vi "Scripting_ConvertSubClassToBaseClass.vi"(0 "SubClass":refnum<vi>, 1 "GOOP4Style":bool, 5 "error in (no error)":errorcluster) -> (19 "error out":errorcluster)   [LabVIEW 2014]
uses:
  <vilib>/Utility/miscctls.llb/LVPositionTypeDef.ctl
  <vilib>/picture/picture.llb/imagedata.ctl
  <resource>/Framework/Providers/Open_GDS/ClassProviders/Provider_EndevoGOOP400/EndevoG4ProviderName.ctl
  <resource>/Framework/Providers/Open_GDS/ClassProviders/Provider_EndevoGOOP400/Templates/EndevoG4TemplateNames.ctl
  <resource>/Framework/Providers/Open_GDS/ClassProviders/Provider_EndevoGOOP300/EndevoProviderName.ctl
  <resource>/Framework/Providers/Open_GDS/ClassProviders/Provider_EndevoGOOP300/Templates/EndevoTemplateNames.ctl
  <resource>/Framework/Providers/Open_GDS/ClassProviders/Provider_LvNativeClass/ClassWriterNative_class/ClassWriterNative.lvclass
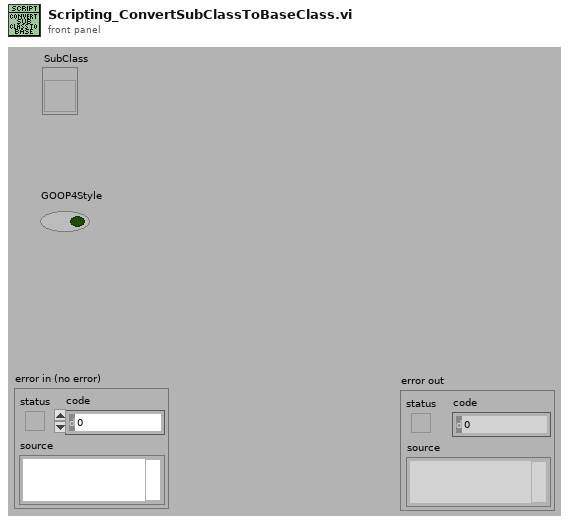
[diagram p1: front panel]
types:
  T1 = cluster{"SubCreate ":path, "ThisSubClass":refnum<vi>, "CurrentBaseClass":refnum<vi>, "SubDestroy":path, "SubKernel":path, "SubAttribute":path, "SubClassAttr":path, "BaseCreate ":path, "BaseDestroy":path, "RootKernel":path, "RootAttribute":path, "RootClassAttr":path, "ThisSubClassName":string, "RootObjectRef":path, "SubObjectRef":path, "AllSubClassFiles":path[], "SubNewVi":path, "ObjectRef":refnum<vi>, "TemplateVersionUsed":string, "BaseNew":path, "Singleton":bool, "AppRef":refnum<vi>}
  T2 = typedef "LVPositionTypeDef.ctl" = cluster{"Left":i32, "Top":i32}
  T3 = typedef "imagedata.ctl" = cluster{"image type":i32, "image depth":i32, "image":u8[], "mask":u8[], "colors":u32[], "Rectangle":cluster{"left":i16, "top":i16, "right":i16, "bottom":i16}}
  T4 = enum32{"invalid VI type", "Standard VI", "Control VI", "Global VI", "Polymorphic VI", "Configuration VI", "SubSystem", "Facade VI", "Method VI"}
  T5 = typedef "EndevoG4TemplateNames.ctl" = enum16{"G4BaseTemplate_Simple_4x4x4", "G4SubTemplate_Simple_4x4x4", "G4BaseTemplate_Simple_6x8x6", "G4SubTemplate_Simple_6x8x6", "G4BaseTemplate_Singleton_4x4x4", "G4SubTemplate_Singleton_4x4x4", "G4BaseTemplate_Singleton_6x8x6", "G4SubTemplate_Singleton_6x8x6", "G4InterfaceTemplate_6x8x6", "G4InterfaceTemplate_4x4x4", "G4BaseTemplate_Simple_5x6x5"}
  T6 = typedef "EndevoG4ProviderName.ctl" = enum16{"EndevoGOOP400"}
  T7 = typedef "EndevoTemplateNames.ctl" = enum16{"BaseTemplate", "SubTemplate", "BaseTemplate_4x4x4", "SubTemplate_4x4x4", "SingletonTemplate"}
  T8 = typedef "EndevoProviderName.ctl" = enum16{"EndevoGOOP300"}
  T9 = typedef "GDSLvCLass_ClassSettingsType.ctl" = cluster{"ClassProviderName":string, "ClassTemplateUsed":string, "ClassTemplateVersion":string, "ClassDescription":string, "PlugIns":T10[], "ConnectorPanePattern":string}
  T10 = typedef "GDSLvClass_PlugIn.ctl" = cluster{"Type":T11, "ID":string, "Version":string, "Path":path, "Name":string, "Data":variant}
  T11 = typedef "GDSLvClass_PlugInTypes.ctl" = enum16{"DesignPattern", "MethodTypes"}
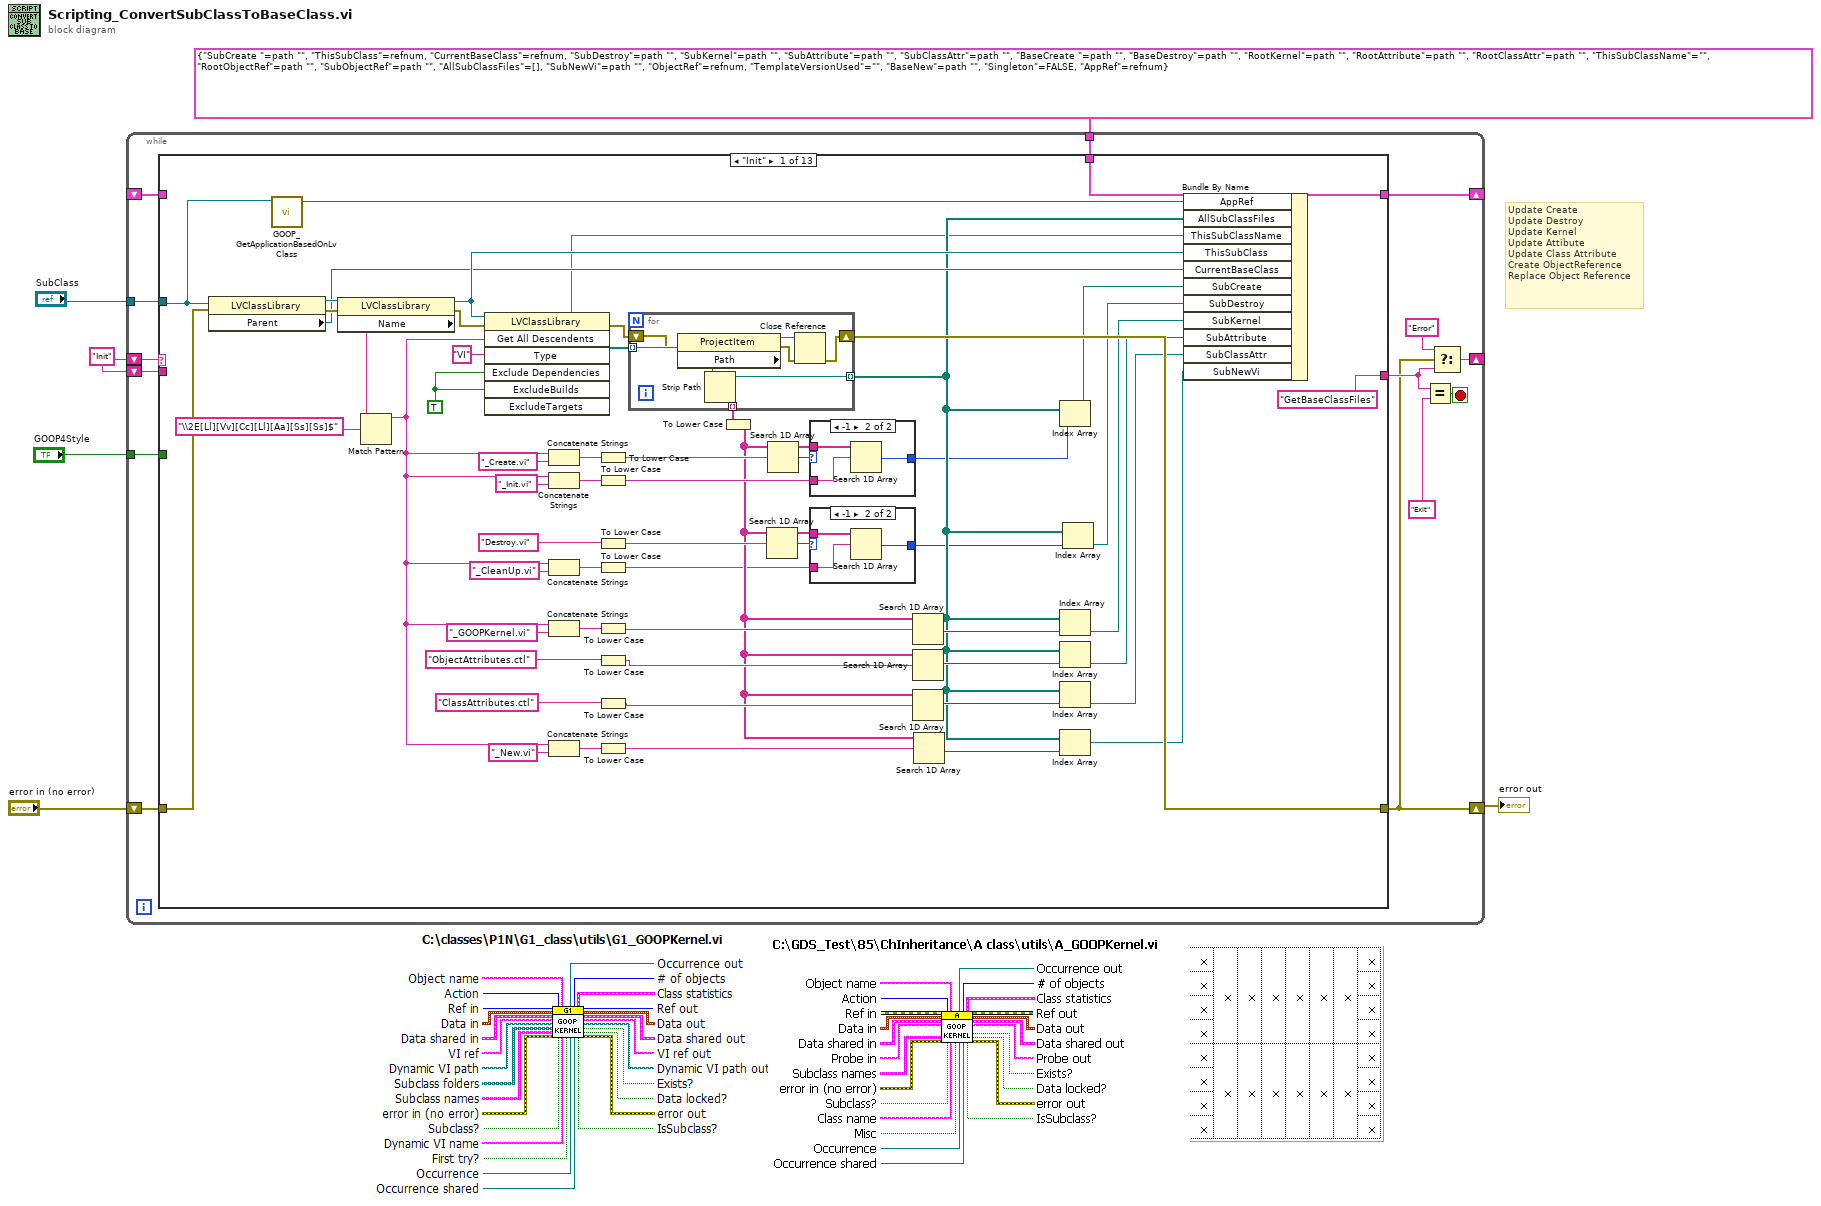
[diagram p0: block diagram]
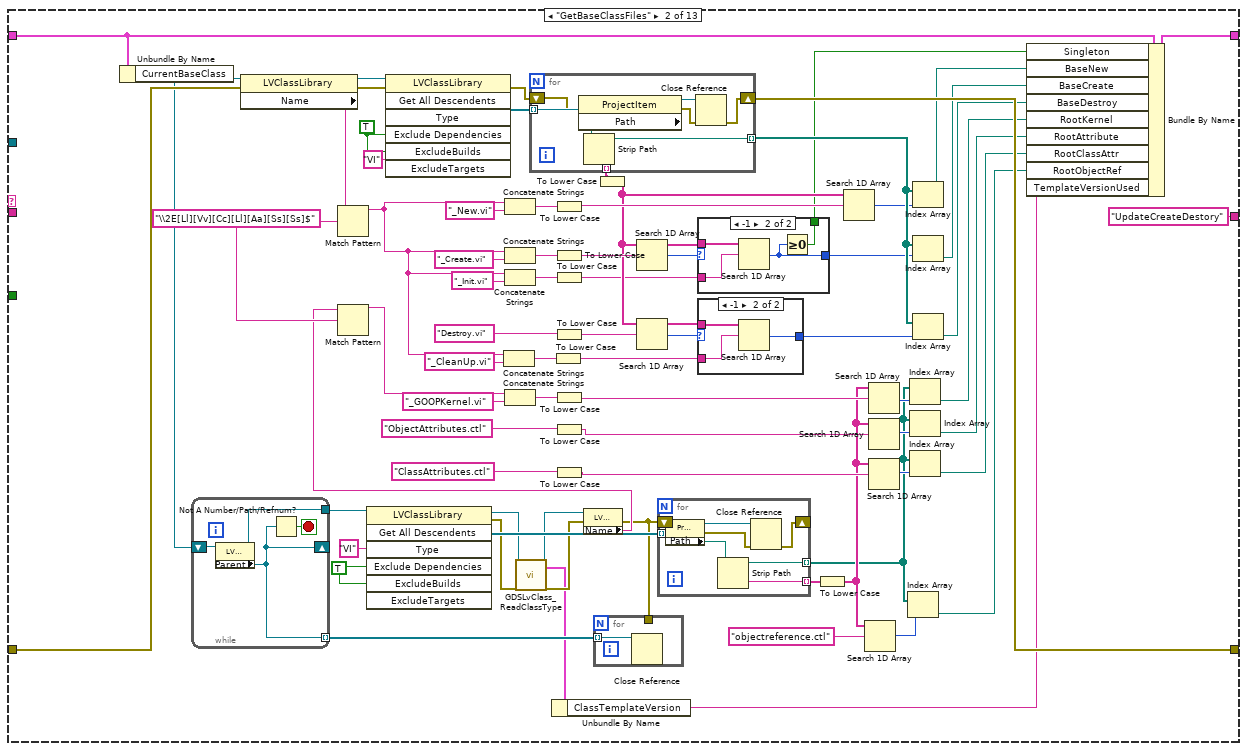
[diagram p4: hidden frame]
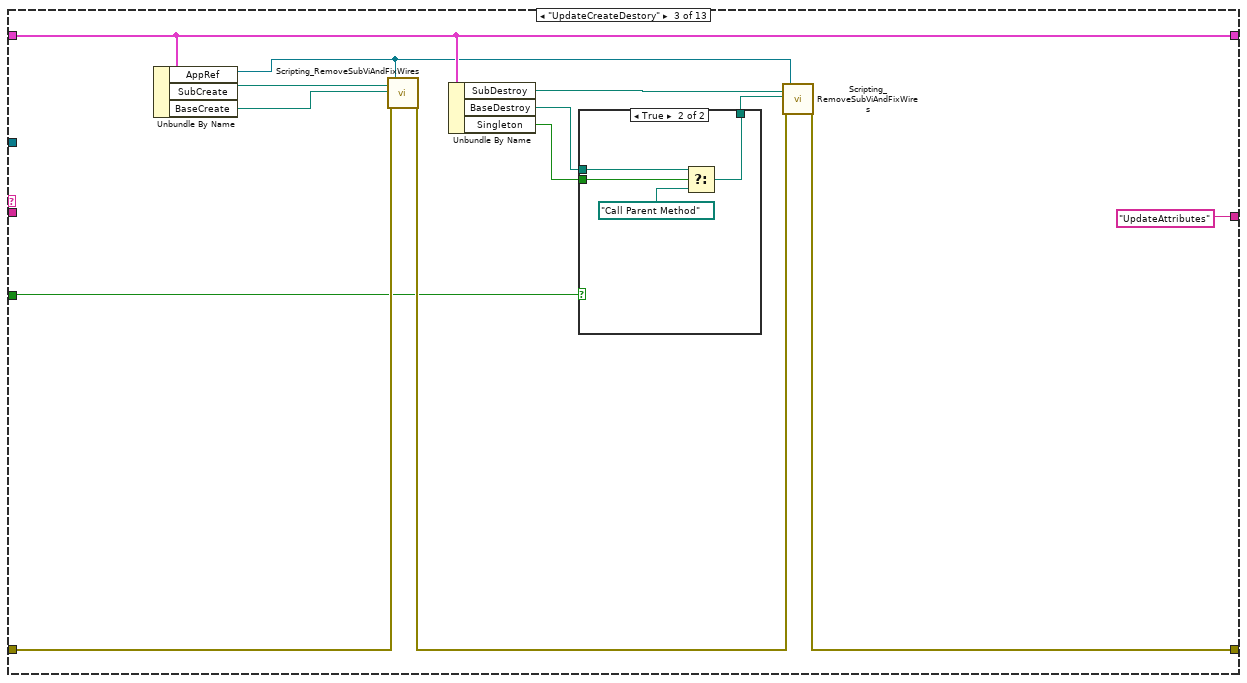
[diagram p7: hidden frame]
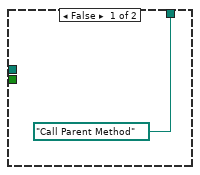
[diagram p8: hidden frame]
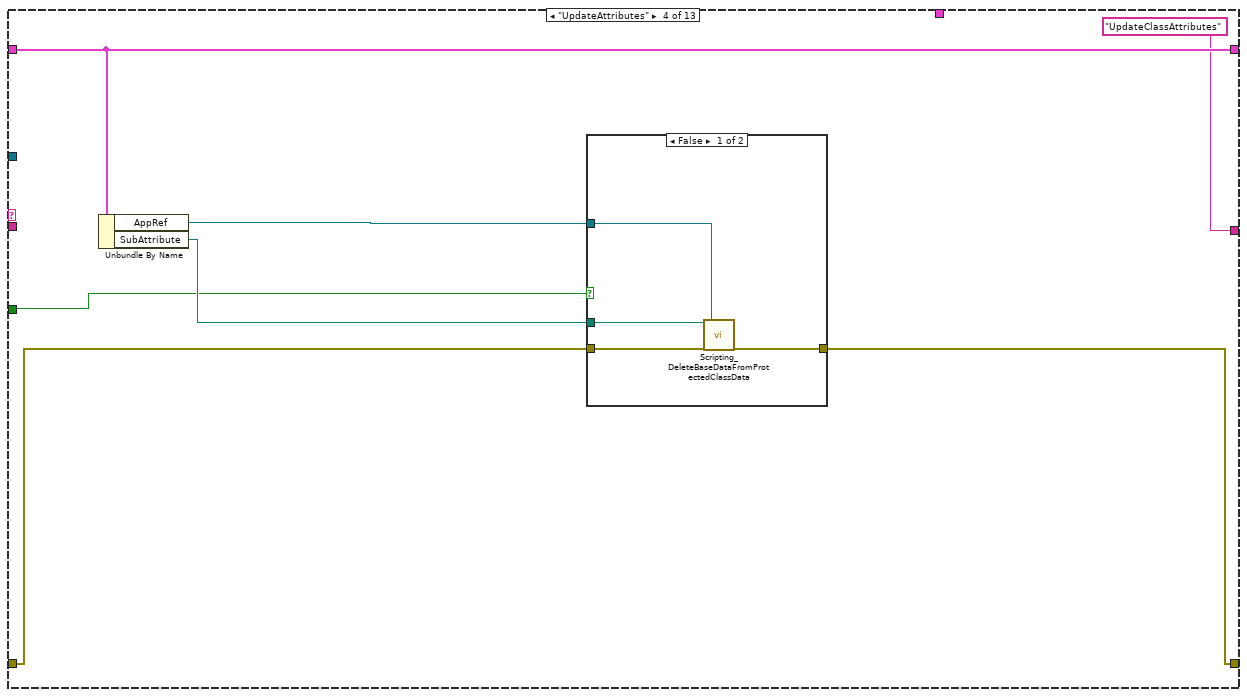
[diagram p9: hidden frame]
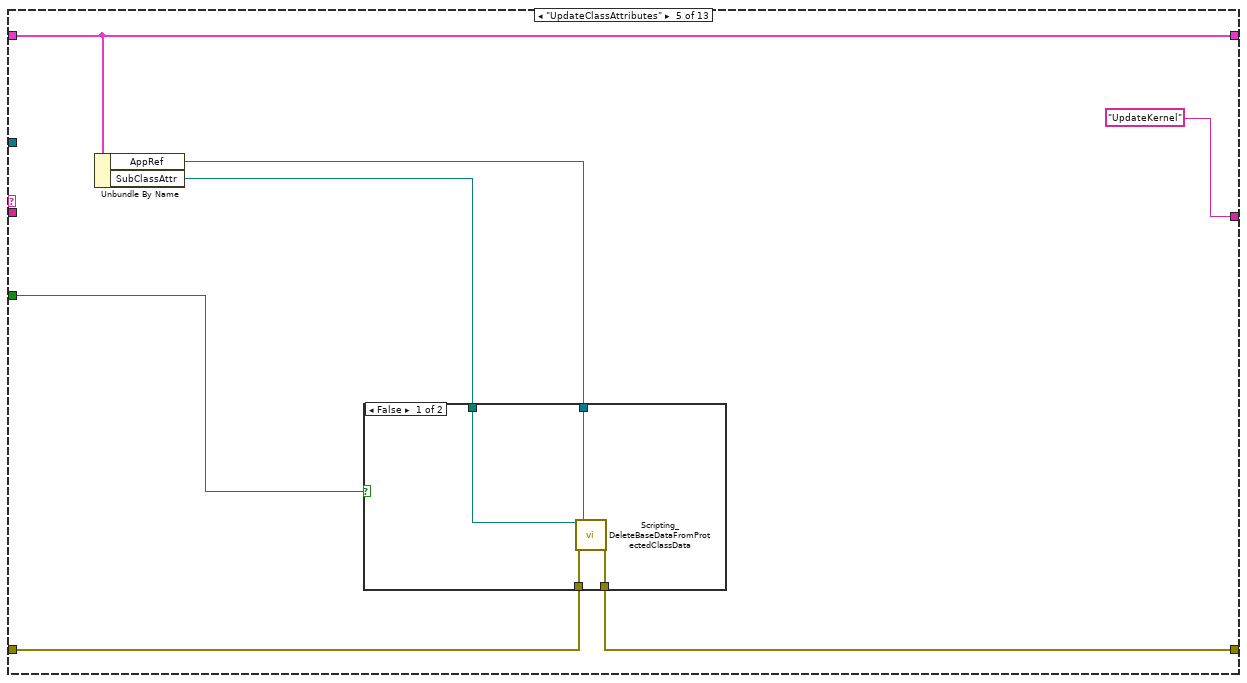
[diagram p11: hidden frame]
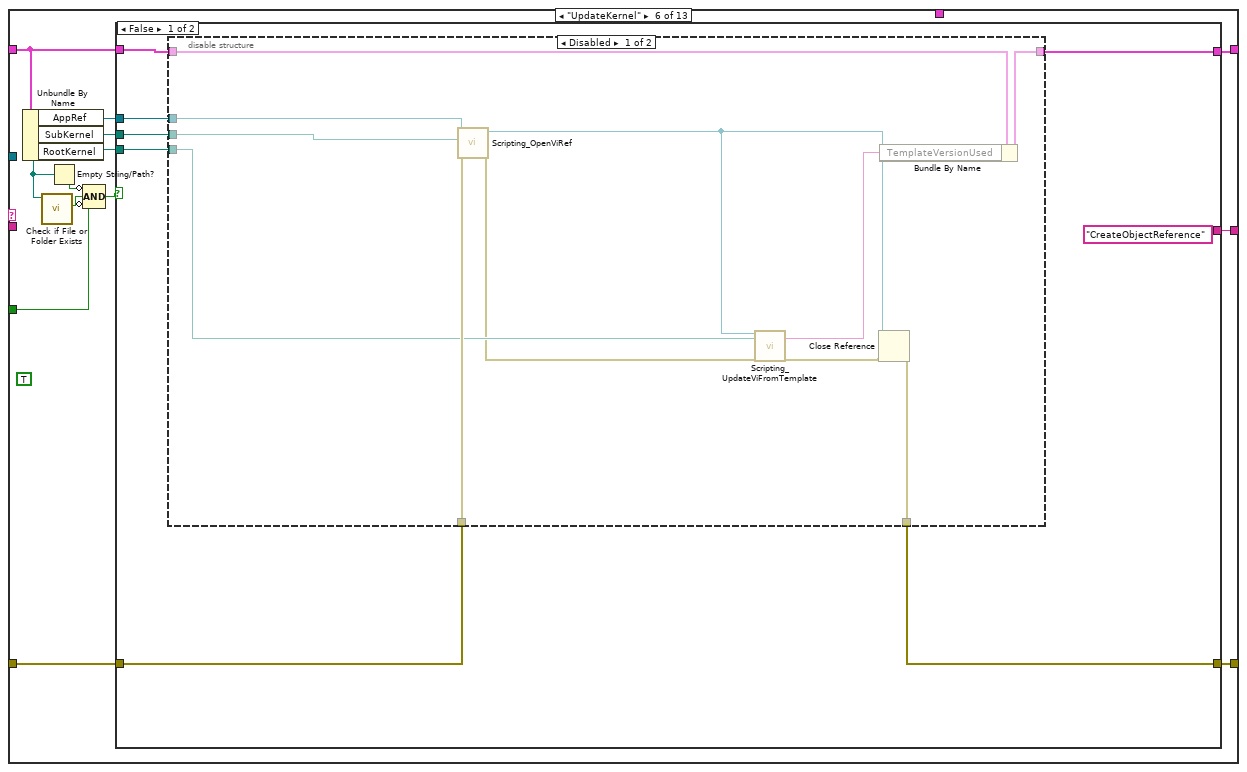
[diagram p13: hidden frame]
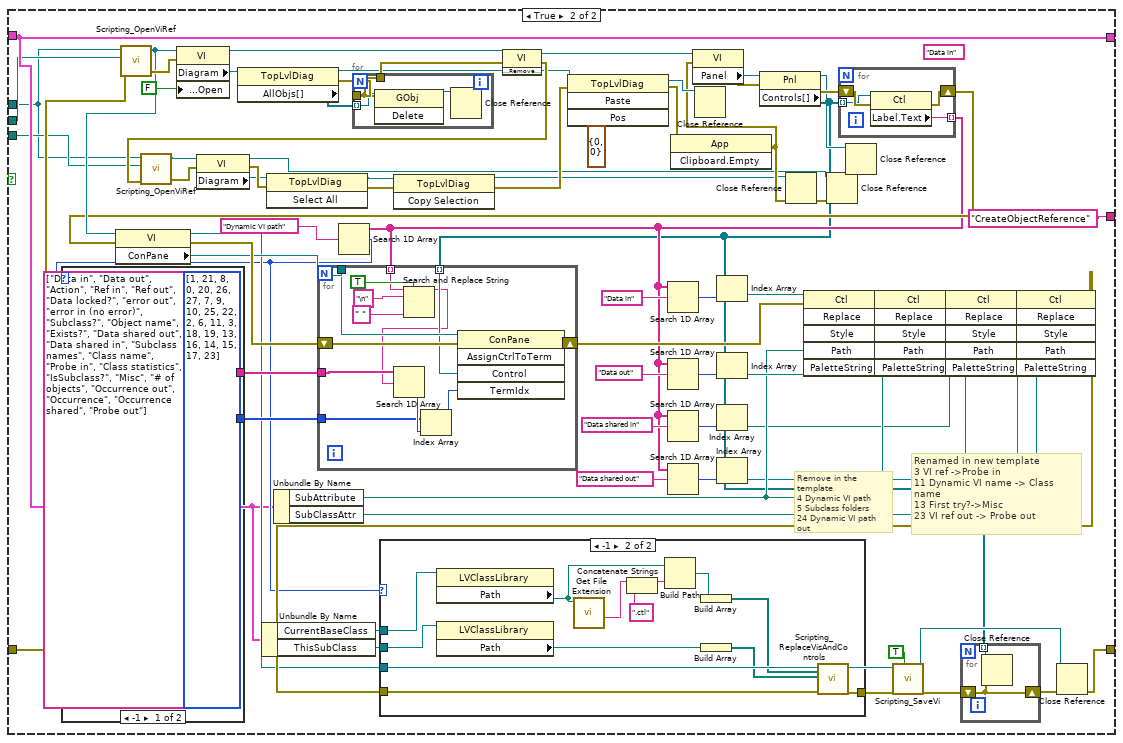
[diagram p15: hidden frame]
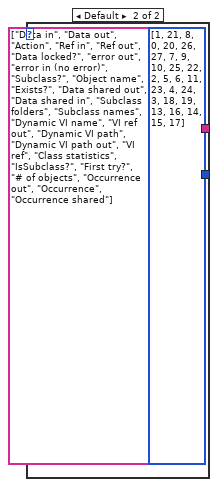
[diagram p17: hidden frame]
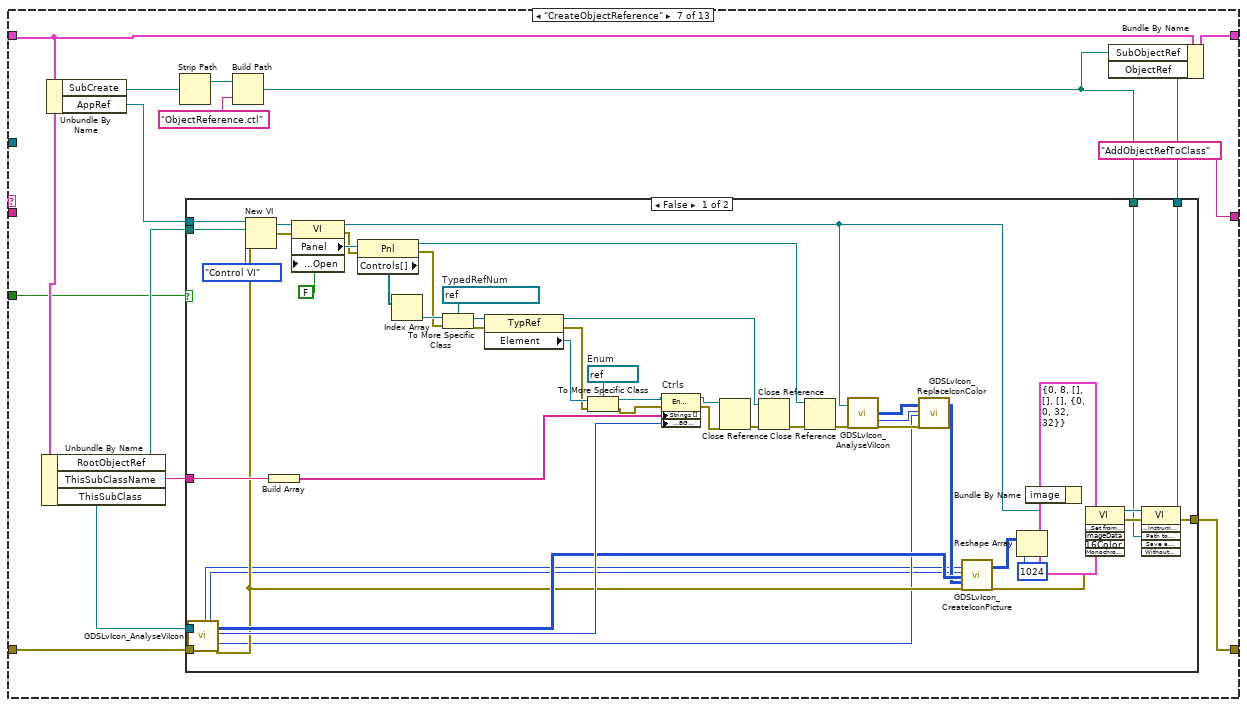
[diagram p18: hidden frame]
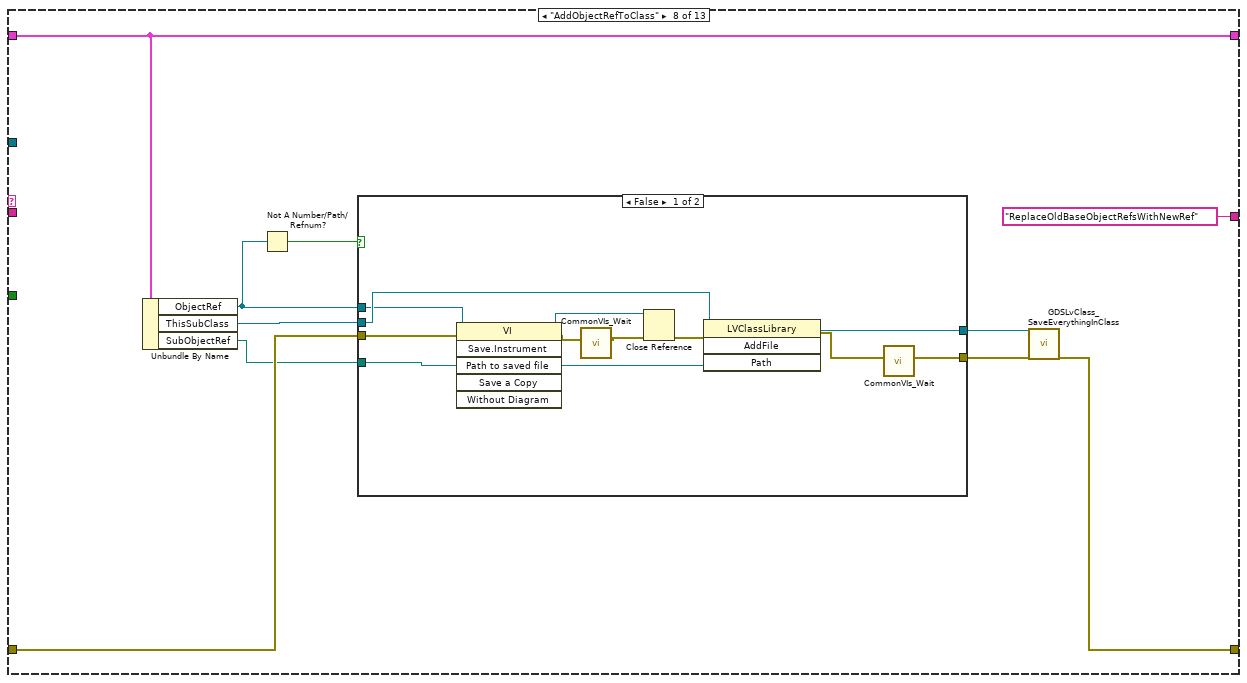
[diagram p20: hidden frame]
diagram:
  w2 = "Init"
  # "Update Create\nUpdate Destroy\nUpdate Kernel\nUpdate Attibute\nUpdate Class Attribute\nCreate ObjectReference\nReplace Object Reference"
  n1 = while {
    shift-right: [w13] -> w5
    shift-left: "error in (no error)" -> [w20]
    shift-right: [w18] -> _
    shift-left: w2 -> [w19]
    shift-right: [w12] -> _
    shift-left: _ -> [w11]
    tunnel: "SubClass" -> [w10]
    tunnel: T1 {"SubCreate "=path "", "ThisSubClass"=refnum, "CurrentBaseClass"=refnum, "SubDestroy"=path "", "SubKernel"=path "", "SubAttribute"=path "", "SubClassAttr"=path "", "BaseCreate "=path "", "BaseDestroy"=path "", "RootKernel"=path "", "RootAttribute"=path "", "RootClassAttr"=path "", "ThisSubClassName"="", "RootObjectRef"=path "", "SubObjectRef"=path "", "AllSubClassFiles"=[], "SubNewVi"=path "", "ObjectRef"=refnum, "TemplateVersionUsed"="", "BaseNew"=path "", "Singleton"=FALSE, "AppRef"=refnum} -> [w9]
    shift-left: w2 -> [w8]
    tunnel: "GOOP4Style" -> [w7]
    stop <- w17 stop-if-true
    n2 = case shown="\"Init\"" w19 {
      tunnel: w20 -> [w45 w136 w204 w218 w229 w247 w390 w457 w485 w538 w578 w588 w597]
      tunnel: [w64 w155 w200 w217 w228 w246 w387 w455 w479 w533 w577 w587 w597] -> w13
      tunnel: ["GetBaseClassFiles" "UpdateCreateDestory" "UpdateAttributes" "UpdateClassAttributes" "UpdateKernel" w248 "AddObjectRefToClass" "ReplaceOldBaseObjectRefsWithNewRef" "RemoveInheritance" "UpdateAllDerivedClasses" "UpdateNEWVI" "CloseReferences" "Exit"] -> w14
      tunnel: [w76 w165 w203 w216 w231 w245 w388 w459 w488 w548 w574 w586 w598] -> w12
      tunnel: w11 -> [_ w137 w203 w216 w231 w244 w385 w459 w488 w548 w574 w586 w598]
      tunnel: w10 -> [w22 _ _ _ _ _ _ _ _ _ w576 _ _]
      tunnel: w9 -> [w44 _ _ _ _ _ _ _ _ _ _ _ _]
      tunnel: w8 -> [_ _ _ _ _ _ _ _ _ _ _ _ w599]
      tunnel: w7 -> [_ _ w198 w214 w226 w238 w383 _ _ w530 w573 w589 _]
      frame "Init" {
        w35 = TRUE ("ExcludeDependencies")
        n3 = property class="LVClassLibrary"(reference=w22, error in=w45) -> (reference out=w72:refnum<vi>, error out=w71:errorcluster, "Parent"=w46:refnum<vi>)
        n4 = call <resource>:"GOOP_GetApplicationBasedOnLvClass.vi"("LVClassLibrary in"=w22) -> ("Application out"=w21:refnum<vi>)  [unwired: 9 in, 1 out]
        n5 = property class="LVClassLibrary"(reference=w72, error in=w71) -> (reference out=w69:refnum<vi>, error out=w70:errorcluster, "Name"=w43:string)
        n6 = Match Pattern(string=w43, regular expression="\\2E[Ll][Vv][Cc][Ll][Aa][Ss][Ss]$") -> (before substring=w25:string)  [unwired: 1 in, 3 out]
        n7 = invoke class="LVClassLibrary" method="Get All Descendents"(reference=w69, error in=w70, "Type"="VI", "Exclude Dependencies"=w35, "ExcludeBuilds"=w35) -> (error out=w73:errorcluster, "All Descendents"=w74:refnum<vi>[])  [unwired: 2 in, 5 out]
        n8 = Concatenate Strings(w25, "_Create.vi" ("string")) -> (w66:string)
        n9 = Concatenate Strings(w25, "_Init.vi" ("string")) -> (w34:string)
        n10 = Concatenate Strings(w25, "_CleanUp.vi" ("string")) -> (w26:string)
        n11 = Concatenate Strings(w25, "_GOOPKernel.vi" ("string")) -> (w60:string)
        n12 = Concatenate Strings(w25, "_New.vi" ("string")) -> (w40:string)
        n13 = To Lower Case(string=w66) -> (all lower case string=w65:string)
        n14 = To Lower Case(string=w34) -> (all lower case string=w31:string)
        n15 = To Lower Case(string="Destroy.vi") -> (all lower case string=w62:string)
        n16 = To Lower Case(string=w26) -> (all lower case string=w23:string)
        n17 = To Lower Case(string=w60) -> (all lower case string=w58:string)
        n18 = To Lower Case(string="ObjectAttributes.ctl") -> (all lower case string=w53:string)
        n19 = To Lower Case(string="ClassAttributes.ctl") -> (all lower case string=w50:string)
        n20 = To Lower Case(string=w40) -> (all lower case string=w41:string)
        n21 = for {
          tunnel: w74 -> [w92] mode=indexing
          shift-right: [w88] -> w64
          shift-left: w73 -> [w89]
          tunnel: [w87] -> w36 mode=indexing
          tunnel: [w86] -> w67 mode=indexing
          n22 = property class="ProjectItem"(reference=w92, error in=w89) -> (reference out=w91:refnum<vi>, error out=w90:errorcluster, "Path"=w87:path)
          n23 = Strip Path(path=w87) -> (name=w86:string)  [unwired: 1 out]
          n24 = Close Reference(reference=w91, error in (no error)=w90) -> (error out=w88:errorcluster)
        }
        n25 = To Lower Case(string=w67) -> (all lower case string=w27:string[])
        n26 = Search 1D Array(1D array=w27, element=w62) -> (index of element=w29:i32)  [unwired: 1 in]
        n27 = Search 1D Array(1D array=w27, element=w65) -> (index of element=w32:i32)  [unwired: 1 in]
        n28 = case shown="-1" w32 {
          selector: w32 -> [w82 _]
          tunnel: w27 -> [_ w85]
          tunnel: w31 -> [_ w84]
          tunnel: [w82 w83] -> w30
          frame 0, Default {
          }
          frame -1 {
            n29 = Search 1D Array(1D array=w85, element=w84) -> (index of element=w83:i32)  [unwired: 1 in]
          }
        }
        n30 = case shown="-1" w29 {
          selector: w29 -> [w78 _]
          tunnel: w27 -> [_ w81]
          tunnel: w23 -> [_ w80]
          tunnel: [w78 w79] -> w28
          frame 0, Default {
          }
          frame -1 {
            n31 = Search 1D Array(1D array=w81, element=w80) -> (index of element=w79:i32)  [unwired: 1 in]
          }
        }
        n32 = Search 1D Array(1D array=w27, element=w58) -> (index of element=w57:i32)  [unwired: 1 in]
        n33 = Search 1D Array(1D array=w27, element=w53) -> (index of element=w52:i32)  [unwired: 1 in]
        n34 = Search 1D Array(1D array=w27, element=w50) -> (index of element=w51:i32)  [unwired: 1 in]
        n35 = Search 1D Array(1D array=w27, element=w41) -> (index of element=w38:i32)  [unwired: 1 in]
        n36 = Index Array(array=w36, index=w30) -> (element=w61:path)
        n37 = Index Array(array=w36, index=w57) -> (element=w49:path)
        n38 = Index Array(array=w36, index=w52) -> (element=w48:path)
        n39 = Index Array(array=w36, index=w51) -> (element=w47:path)
        n40 = Index Array(array=w36, index=w38) -> (element=w37:path)
        n41 = Index Array(array=w36, index=w28) -> (element=w56:path)
        n42 = Bundle By Name(cluster=w44, "AppRef"=w21, "AllSubClassFiles"=w36, "ThisSubClassName"=w25, "ThisSubClass"=w69, "CurrentBaseClass"=w46, "SubCreate"=w61, "SubDestroy"=w56, "SubKernel"=w49, "SubAttribute"=w48, "SubClassAttr"=w47, "SubNewVi"=w37) -> (w76:T1)
      }
      frame "GetBaseClassFiles" {
        w118 = TRUE ("ExcludeDependencies")
        w119 = TRUE ("ExcludeDependencies")
        w128 = "\\2E[Ll][Vv][Cc][Ll][Aa][Ss][Ss]$" ("regular expression")
        n43 = Unbundle By Name(w137) -> ("CurrentBaseClass"=w134:refnum<vi>)
        n44 = while {
          shift-right: [w185] -> _
          shift-left: w134 -> [w186]
          tunnel: [w185] -> w133 mode=indexing
          tunnel: [w184] -> w131
          stop <- w187 stop-if-true
          n45 = property class="LVClassLibrary"(reference=w186) -> (reference out=w184:refnum<vi>, "Parent"=w185:refnum<vi>)  [unwired: 1 in, 1 out]
          n46 = Not A Number/Path/Refnum?(number/path/refnum=w185) -> (NaN/Path/Refnum?=w187:bool)
        }
        n47 = property class="LVClassLibrary"(reference=w134, error in=w136) -> (reference out=w160:refnum<vi>, error out=w161:errorcluster, "Name"=w135:string)
        n48 = Match Pattern(string=w135, regular expression=w128) -> (before substring=w96:string)  [unwired: 1 in, 3 out]
        n49 = invoke class="LVClassLibrary" method="Get All Descendents"(reference=w131, "Type"="VI", "Exclude Dependencies"=w119, "ExcludeBuilds"=w119) -> (reference out=w117:refnum<vi>, error out=w115:errorcluster, "All Descendents"=w130:refnum<vi>[])  [unwired: 3 in, 4 out]
        n50 = invoke class="LVClassLibrary" method="Get All Descendents"(reference=w160, error in=w161, "Type"="VI", "Exclude Dependencies"=w118, "ExcludeBuilds"=w118) -> (error out=w162:errorcluster, "All Descendents"=w163:refnum<vi>[])  [unwired: 2 in, 5 out]
        n51 = Concatenate Strings(w96, "_CleanUp.vi" ("string")) -> (w98:string)
        n52 = Concatenate Strings(w96, "_New.vi" ("string")) -> (w111:string)
        n53 = Concatenate Strings(w96, "_Create.vi" ("string")) -> (w157:string)
        n54 = Concatenate Strings(w96, "_Init.vi" ("string")) -> (w100:string)
        n55 = call <resource>:"GDSLvClass_ReadClassType.vi"("Class Refnum In"=w117, "error in (no error)"=w115) -> ("Class Refnum Out"=w116:refnum<vi>, "ClassSettings"=w113:T9, "error out"=w114:errorcluster)  [unwired: 15 in]
        n56 = for {
          tunnel: w163 -> [w194] mode=indexing
          shift-right: [w190] -> w155
          shift-left: w162 -> [w191]
          tunnel: [w189] -> w108 mode=indexing
          tunnel: [w188] -> w158 mode=indexing
          n57 = property class="ProjectItem"(reference=w194, error in=w191) -> (reference out=w193:refnum<vi>, error out=w192:errorcluster, "Path"=w189:path)
          n58 = Strip Path(path=w189) -> (name=w188:string)  [unwired: 1 out]
          n59 = Close Reference(reference=w193, error in (no error)=w192) -> (error out=w190:errorcluster)
        }
        n60 = Unbundle By Name(w113) -> ("ClassTemplateVersion"=w112:string)
        n61 = To Lower Case(string=w98) -> (all lower case string=w94:string)
        n62 = To Lower Case(string=w111) -> (all lower case string=w109:string)
        n63 = To Lower Case(string=w157) -> (all lower case string=w156:string)
        n64 = To Lower Case(string=w100) -> (all lower case string=w95:string)
        n65 = To Lower Case(string="Destroy.vi") -> (all lower case string=w153:string)
        n66 = To Lower Case(string="ObjectAttributes.ctl") -> (all lower case string=w144:string)
        n67 = To Lower Case(string="ClassAttributes.ctl") -> (all lower case string=w141:string)
        n68 = property class="LVClassLibrary"(reference=w116, error in=w114) -> (error out=w120:errorcluster, "Name"=w126:string)  [unwired: 1 out]
        n69 = Match Pattern(string=w126, regular expression=w128) -> (before substring=w127:string)  [unwired: 1 in, 3 out]
        n70 = Concatenate Strings(w127, "_GOOPKernel.vi" ("string")) -> (w151:string)
        n71 = To Lower Case(string=w151) -> (all lower case string=w149:string)
        n72 = for {
          tunnel: w133 -> [w183] mode=indexing
          tunnel: w120 -> [_]
          n73 = Close Reference(reference=w183) -> ()  [unwired: 1 in, 1 out]
        }
        n74 = To Lower Case(string=w158) -> (all lower case string=w101:string[])
        n75 = Search 1D Array(1D array=w101, element=w156) -> (index of element=w104:i32)  [unwired: 1 in]
        n76 = Search 1D Array(1D array=w101, element=w153) -> (index of element=w105:i32)  [unwired: 1 in]
        n77 = for {
          tunnel: w130 -> [w182] mode=indexing
          shift-right: [w178] -> _
          shift-left: w120 -> [w179]
          tunnel: [w177] -> w122 mode=indexing
          tunnel: [w176] -> w129 mode=indexing
          n78 = property class="ProjectItem"(reference=w182, error in=w179) -> (reference out=w181:refnum<vi>, error out=w180:errorcluster, "Path"=w177:path)
          n79 = Strip Path(path=w177) -> (name=w176:string)  [unwired: 1 out]
          n80 = Close Reference(reference=w181, error in (no error)=w180) -> (error out=w178:errorcluster)
        }
        n81 = case shown="-1" w104 {
          selector: w104 -> [w171 _]
          tunnel: w101 -> [_ w175]
          tunnel: w95 -> [_ w174]
          tunnel: [w171 w173] -> w103
          tunnel: [_ w172] -> w93
          frame 0, Default {
          }
          frame -1 {
            n82 = Search 1D Array(1D array=w175, element=w174) -> (index of element=w173:i32)  [unwired: 1 in]
            n83 = Greater Or Equal To 0?(x=w173) -> (x >= 0?=w172:bool)
          }
        }
        n84 = case shown="-1" w105 {
          selector: w105 -> [w167 _]
          tunnel: w101 -> [_ w170]
          tunnel: w94 -> [_ w169]
          tunnel: [w167 w168] -> w102
          frame 0, Default {
          }
          frame -1 {
            n85 = Search 1D Array(1D array=w170, element=w169) -> (index of element=w168:i32)  [unwired: 1 in]
          }
        }
        n86 = To Lower Case(string=w129) -> (all lower case string=w123:string[])
        n87 = Search 1D Array(1D array=w101, element=w109) -> (index of element=w107:i32)  [unwired: 1 in]
        n88 = Search 1D Array(1D array=w123, element="objectreference.ctl") -> (index of element=w124:i32)  [unwired: 1 in]
        n89 = Search 1D Array(1D array=w123, element=w149) -> (index of element=w148:i32)  [unwired: 1 in]
        n90 = Search 1D Array(1D array=w123, element=w144) -> (index of element=w143:i32)  [unwired: 1 in]
        n91 = Search 1D Array(1D array=w123, element=w141) -> (index of element=w142:i32)  [unwired: 1 in]
        n92 = Index Array(array=w122, index=w124) -> (element=w121:path)
        n93 = Index Array(array=w122, index=w148) -> (element=w140:path)
        n94 = Index Array(array=w122, index=w143) -> (element=w139:path)
        n95 = Index Array(array=w122, index=w142) -> (element=w138:path)
        n96 = Index Array(array=w108, index=w107) -> (element=w106:path)
        n97 = Index Array(array=w108, index=w103) -> (element=w152:path)
        n98 = Index Array(array=w108, index=w102) -> (element=w147:path)
        n99 = Bundle By Name(cluster=w137, "Singleton"=w93, "BaseNew"=w106, "BaseCreate"=w152, "BaseDestroy"=w147, "RootKernel"=w140, "RootAttribute"=w139, "RootClassAttr"=w138, "RootObjectRef"=w121, "TemplateVersionUsed"=w112) -> (w165:T1)
      }
      frame "UpdateCreateDestory" {
        n100 = Unbundle By Name(w203) -> ("AppRef"=w195:refnum<vi>, "SubCreate"=w206:path, "BaseCreate"=w205:path)
        n101 = call <resource>:"Scripting_RemoveSubViAndFixWires.vi"("MainViPath/ViRef/BlockDiagramRef"=w206, "SubVIToRemove"=w205, "error in (no error)"=w204, "AppRef"=w195) -> ("error out"=w201:errorcluster)  [unwired: 15 in]
        n102 = Unbundle By Name(w203) -> ("SubDestroy"=w202:path, "BaseDestroy"=w196:path, "Singleton"=w197:bool)
        n103 = case shown="True" w198 {
          tunnel: [path "Call Parent Method" ("SubVIToRemove") w209] -> w199
          tunnel: w197 -> [_ w212]
          tunnel: w196 -> [_ w210]
          frame False {
          }
          frame True {
            n104 = Select(t=w210, s=w212, f=path "Call Parent Method" ("SubVIToRemove")) -> (s? t:f=w209:path)
          }
        }
        n105 = call <resource>:"Scripting_RemoveSubViAndFixWires.vi"("MainViPath/ViRef/BlockDiagramRef"=w202, "SubVIToRemove"=w199, "error in (no error)"=w201, "AppRef"=w195) -> ("error out"=w200:errorcluster)  [unwired: 15 in]
      }
      frame "UpdateAttributes" {
        n106 = Unbundle By Name(w216) -> ("AppRef"=w213:refnum<vi>, "SubAttribute"=w219:path)
        n107 = case shown="False" w214 {
          tunnel: w219 -> [w223 _]
          tunnel: w218 -> [w222 w224]
          tunnel: [w221 w224] -> w217
          tunnel: w213 -> [w220 _]
          frame False {
            n108 = call <resource>:"Scripting_DeleteBaseDataFromProtectedClassData.vi"("SubAttribute"=w223, "error in (no error)"=w222, "AppRef"=w220) -> ("error out"=w221:errorcluster)  [unwired: 16 in]
          }
          frame True {
          }
        }
      }
      frame "UpdateClassAttributes" {
        n109 = Unbundle By Name(w231) -> ("AppRef"=w225:refnum<vi>, "SubClassAttr"=w227:path)
        n110 = case shown="False" w226 {
          tunnel: w229 -> [w235 w236]
          tunnel: [w234 w236] -> w228
          tunnel: w227 -> [w233 _]
          tunnel: w225 -> [w232 _]
          frame False {
            n111 = call <resource>:"Scripting_DeleteBaseDataFromProtectedClassData.vi"("SubAttribute"=w233, "error in (no error)"=w235, "AppRef"=w232) -> ("error out"=w234:errorcluster)  [unwired: 16 in]
          }
          frame True {
          }
        }
      }
      frame "UpdateKernel" {
        (unwired) TRUE
        n112 = Unbundle By Name(w244) -> ("AppRef"=w237:refnum<vi>, "SubKernel"=w242:path, "RootKernel"=w243:path)
        n113 = call <vilib>:"Check if File or Folder Exists.vi"("path"=w242) -> ("file or folder exists?"=w239:bool)  [unwired: 8 in, 2 out]
        n114 = Empty String/Path?(string/path=w242) -> (empty?=w241:bool)
        n115 = Compound Arithmetic op=AND(invert w241, w239, invert w238) -> (w240:bool)
        n116 = case shown="False" w240 {
          tunnel: ["CreateObjectReference" "CreateObjectReference"] -> w248
          tunnel: w247 -> [w253 w315]
          tunnel: w244 -> [w255 w275]
          tunnel: [w252 w283] -> w246
          tunnel: [w254 w275] -> w245
          tunnel: w242 -> [w251 w272]
          tunnel: w243 -> [w250 w271]
          tunnel: w237 -> [w249 w270]
          frame False {
            n117 = disable-structure shown="Disabled" {
              disable-tunnel: w255 -> [w266 w268]
              disable-tunnel: [w265 w268] -> w254
              disable-tunnel: w253 -> [w264 w269]
              disable-tunnel: [w263 w269] -> w252
              disable-tunnel: w251 -> [w262 _]
              disable-tunnel: w250 -> [w261 _]
              disable-tunnel: w249 -> [w257 _]
              frame Disabled {
                n118 = call <resource>:"Scripting_OpenViRef.vi"("error in"=w264, "ViPath/ViName/Viref"=w262, "AppRef"=w257) -> ("error out"=w260:errorcluster, "vi reference"=w258:refnum<vi>)  [unwired: 6 in, 1 out]
                n119 = call <resource>:"Scripting_UpdateViFromTemplate.vi"("ViRef"=w258, "TemplateVI(Path or Ref)"=w261, "error in (no error)"=w260) -> ("TemplateVersionUsed"=w267:string, "error out"=w259:errorcluster)  [unwired: 15 in]
                n120 = Close Reference(reference=w258, error in (no error)=w259) -> (error out=w263:errorcluster)
                n121 = Bundle By Name(cluster=w266, "TemplateVersionUsed"=w267) -> (w265:T1)
              }
              frame Enabled {
              }
            }
          }
          frame True {
            (unwired) "Data in" ("Label.Text")
            # "Renamed in new template\n3 VI ref ->Probe in\n11 Dynamic VI name -> Class name\n13 First try?->Misc\n23 VI ref out -> Probe out"
            # "Remove in the template\n4 Dynamic VI path\n5 Subclass folders\n24 Dynamic VI path out"
            n122 = call <resource>:"Scripting_OpenViRef.vi"("error in"=w315, "ViPath/ViName/Viref"=w272, "AppRef"=w270) -> ("error out"=w340:errorcluster, "vi reference"=w329:refnum<vi>)  [unwired: 6 in, 1 out]
            n123 = property class="VI"(reference=w329, error in=w340, "Front Panel.Open"=FALSE ("Front Panel Window:Open")) -> (reference out=w324:refnum<vi>, "Diagram"=w327:refnum<vi>)  [unwired: 1 out]
            n124 = property class="TopLvlDiag"(reference=w327) -> (reference out=w320:refnum<vi>, error out=w326:errorcluster, "AllObjs[]"=w325:refnum<vi>[])  [unwired: 1 in]
            n125 = Unbundle By Name(w275) -> ("CurrentBaseClass"=w274:refnum<vi>, "ThisSubClass"=w273:refnum<vi>)
            n126 = Unbundle By Name(w275) -> ("SubAttribute"=w302:path, "SubClassAttr"=w297:path)
            n127 = for {
              tunnel: w326 -> [w375]
              tunnel: w325 -> [w376] mode=indexing
              tunnel: [w375] -> w323
              n128 = invoke class="GObj" method="Delete"(reference=w376, error in=w375) -> (reference out=w377:refnum<vi>)  [unwired: 1 in, 2 out]
              n129 = Close Reference(reference=w377) -> ()  [unwired: 1 in, 1 out]
            }
            n130 = invoke class="VI" method="BD.Remove Bad Wires"(reference=w324, error in=w323) -> (reference out=w319:refnum<vi>, error out=w322:errorcluster)  [unwired: 1 in, 1 out]
            n131 = call <resource>:"Scripting_OpenViRef.vi"("error in"=w322, "ViPath/ViName/Viref"=w271, "AppRef"=w270) -> ("error out"=w335:errorcluster, "vi reference"=w334:refnum<vi>)  [unwired: 6 in, 1 out]
            n132 = property class="VI"(reference=w334, error in=w335) -> (reference out=w290:refnum<vi>, error out=w339:errorcluster, "Diagram"=w336:refnum<vi>)
            n133 = invoke class="TopLvlDiag" method="Select All"(reference=w336, error in=w339) -> (reference out=w337:refnum<vi>, error out=w338:errorcluster)  [unwired: 1 in, 1 out]
            n134 = invoke class="TopLvlDiag" method="Copy Selection"(reference=w337, error in=w338) -> (reference out=w292:refnum<vi>, error out=w321:errorcluster)  [unwired: 1 in, 1 out]
            n135 = invoke class="TopLvlDiag" method="Paste"(reference=w320, error in=w321, "Pos"=T2 {"Left"=0, "Top"=0} ("Position")) -> (reference out=w295:refnum<vi>, error out=w296:errorcluster)  [unwired: 1 in, 2 out]
            n136 = invoke class="App" method="Clipboard.Empty"(error in=w296) -> (error out=w293:errorcluster)  [unwired: 2 in, 2 out]
            n137 = property class="VI"(reference=w319, error in=w293) -> (error out=w331:errorcluster, "Panel"=w332:refnum<vi>)  [unwired: 1 out]
            n138 = Close Reference(reference=w295) -> ()  [unwired: 1 in, 1 out]
            n139 = property class="Pnl"(reference=w332, error in=w331) -> (reference out=w294:refnum<vi>, error out=w330:errorcluster, "Controls[]"=w280:refnum<vi>[])
            n140 = Close Reference(reference=w292, error in (no error)=w293) -> (error out=w291:errorcluster)
            n141 = Close Reference(reference=w290, error in (no error)=w291) -> ()  [unwired: 1 out]
            n142 = for {
              tunnel: w280 -> [w378] mode=indexing
              shift-right: [w380] -> w328
              shift-left: w330 -> [w381]
              tunnel: [w379] -> w285 mode=indexing
              n143 = property class="Ctl"(reference=w378, error in=w381) -> (error out=w380:errorcluster, "Label.Text"=w379:string)  [unwired: 1 out]
            }
            n144 = property class="VI"(reference=w329, error in=w328) -> (reference out=w277:refnum<vi>, error out=w316:errorcluster, "ConPane"=w282:refnum<vi>)
            n145 = Search 1D Array(1D array=w285, element="Dynamic VI path" ("Id")) -> (index of element=w276:i32)  [unwired: 1 in]
            n146 = case shown="-1" w276 {
              tunnel: [string[] ["Data in", "Data out", "Action", "Ref in", "Ref out", "Data locked?", "error out", "error in (no error)", "Subclass?", "Object name", "Exists?", "Data shared out", "Data shared in", "Subclass names", "Class name", "Probe in", "Class statistics", "IsSubclass?", "Misc", "# of objects", "Occurrence out", "Occurrence", "Occurrence shared", "Probe out"] ("Array") string[] ["Data in", "Data out", "Action", "Ref in", "Ref out", "Data locked?", "error out", "error in (no error)", "Subclass?", "Object name", "Exists?", "Data shared out", "Data shared in", "Subclass folders", "Subclass names", "Dynamic VI name", "VI ref out", "Dynamic VI path", "Dynamic VI path out", "VI ref", "Class statistics", "IsSubclass?", "First try?", "# of objects", "Occurrence out", "Occurrence", "Occurrence shared"] ("Array")] -> w318
              tunnel: [i32[] [1, 21, 8, 0, 20, 26, 27, 7, 9, 10, 25, 22, 2, 6, 11, 3, 18, 19, 13, 16, 14, 15, 17, 23] i32[] [1, 21, 8, 0, 20, 26, 27, 7, 9, 10, 25, 22, 2, 5, 6, 11, 23, 4, 24, 3, 18, 19, 13, 16, 14, 15, 17]] -> w317
              frame -1 {
              }
              frame Default {
              }
            }
            n147 = for {
              tunnel: w285 -> [w361] mode=indexing
              tunnel: w282 -> [w372]
              tunnel: w318 -> [w365]
              tunnel: w280 -> [w366] mode=indexing
              tunnel: w317 -> [w370]
              shift-right: [w367] -> w310
              shift-left: w316 -> [w368]
              n148 = Search and Replace String(replace all?=TRUE ("replace all? (F)"), input string=w361, search string="\n", replace string=" " ("replace string (\"\")")) -> (result string=w360:string)  [unwired: 4 in, 3 out]
              n149 = Search 1D Array(1D array=w365, element=w360) -> (index of element=w371:i32)  [unwired: 1 in]
              n150 = Index Array(array=w370, index=w371) -> (element=w369:i32)
              n151 = invoke class="ConPane" method="AssignCtrlToTerm"(reference=w372, error in=w368, "Control"=w366, "TermIdx"=w369) -> (error out=w367:errorcluster)  [unwired: 1 in, 4 out]
            }
            n152 = Search 1D Array(1D array=w285, element="Data in" ("Label.Text")) -> (index of element=w314:i32)  [unwired: 1 in]
            n153 = Search 1D Array(1D array=w285, element="Data out" ("Label.Text")) -> (index of element=w309:i32)  [unwired: 1 in]
            n154 = Search 1D Array(1D array=w285, element="Data shared in" ("Label.Text")) -> (index of element=w308:i32)  [unwired: 1 in]
            n155 = Search 1D Array(1D array=w285, element="Data shared out" ("Label.Text")) -> (index of element=w307:i32)  [unwired: 1 in]
            n156 = Index Array(array=w280, index=w314) -> (element=w312:refnum<vi>)
            n157 = Index Array(array=w280, index=w309) -> (element=w303:refnum<vi>)
            n158 = Index Array(array=w280, index=w308) -> (element=w299:refnum<vi>)
            n159 = Index Array(array=w280, index=w307) -> (element=w298:refnum<vi>)
            n160 = invoke class="Ctl" method="Replace"(reference=w312, error in=w310, "Path"=w302) -> (error out=w311:errorcluster)  [unwired: 3 in, 5 out]
            n161 = Close Reference(reference=w294) -> ()  [unwired: 1 in, 1 out]
            n162 = invoke class="Ctl" method="Replace"(reference=w303, error in=w311, "Path"=w302) -> (error out=w300:errorcluster)  [unwired: 3 in, 5 out]
            n163 = invoke class="Ctl" method="Replace"(reference=w299, error in=w300, "Path"=w297) -> (error out=w301:errorcluster)  [unwired: 3 in, 5 out]
            n164 = invoke class="Ctl" method="Replace"(reference=w298, error in=w301, "Path"=w297) -> (error out=w279:errorcluster)  [unwired: 3 in, 5 out]
            n165 = case shown="-1" w276 {
              tunnel: w277 -> [_ w355]
              tunnel: w279 -> [w342 w354]
              tunnel: [w342 w353] -> w278
              tunnel: w274 -> [_ w350]
              tunnel: w273 -> [_ w349]
              frame Default {
              }
              frame -1 {
                n166 = property class="LVClassLibrary"(reference=w350) -> ("Path"=w346:path)  [unwired: 1 in, 2 out]
                n167 = property class="LVClassLibrary"(reference=w349) -> ("Path"=w348:path)  [unwired: 1 in, 2 out]
                n168 = call <vilib>:"Get File Extension.vi"("file"=w346) -> ("filename without extension"=w345:string)  [unwired: 7 in, 3 out]
                n169 = Concatenate Strings(w345, ".ctl" ("string")) -> (w344:string)
                n170 = Build Path(base path=w346, name or relative path=w344) -> (appended path=w347:path)
                n171 = Build Array(w347) -> (w352:path[])
                n172 = Build Array(w348) -> (w351:path[])
                n173 = call <resource>:"Scripting_ReplaceVisAndControls.vi"("ViRef"=w355, "OldVIsAndControls"=w352, "NewVIsAndControls"=w351, "error in (no error)"=w354) -> ("error out"=w353:errorcluster)  [unwired: 14 in, 1 out]
              }
            }
            n174 = call <resource>:"Scripting_SaveVi.vi"("ForceResaving(False)"=TRUE, "error in (no error)"=w278, "VIRefToSaveIn"=w277) -> ("error out"=w287:errorcluster, "VIRefToSaveOut"=w288:refnum<vi>)  [unwired: 7 in]
            n175 = for {
              tunnel: w280 -> [w374] mode=indexing
              shift-right: [w373] -> w289
              shift-left: w287 -> [w373]
              n176 = Close Reference(reference=w374, error in (no error)=w373) -> ()  [unwired: 1 out]
            }
            n177 = Close Reference(reference=w288, error in (no error)=w289) -> (error out=w283:errorcluster)
          }
        }
      }
      frame "CreateObjectReference" {
        n178 = Unbundle By Name(w385) -> ("RootObjectRef"=w391:path, "ThisSubClassName"=w394:string, "ThisSubClass"=w389:refnum<vi>)
        n179 = Unbundle By Name(w385) -> ("SubCreate"=w393:path, "AppRef"=w382:refnum<vi>)
        n180 = Strip Path(path=w393) -> (stripped path=w396:path)  [unwired: 1 out]
        n181 = Build Path(base path=w396, name or relative path="ObjectReference.ctl") -> (appended path=w384:path)
        n182 = case shown="False" w383 {
          tunnel: w394 -> [w446 _]
          tunnel: w391 -> [w445 _]
          tunnel: w390 -> [w414 w449]
          tunnel: w389 -> [w413 _]
          tunnel: [w400 w449] -> w387
          tunnel: [w399 _] -> w386
          tunnel: w384 -> [w398 _]
          tunnel: w382 -> [w397 _]
          frame False {
            w434 = refnum<vi> refnum  # Enum
            w439 = refnum<vi> refnum  # TypedRefNum
            n183 = call <resource>:"GDSLvIcon_AnalyseViIcon.vi"("ViRef/LvCLassRef/LvLibRef/ViPath"=w413, "error in (no error)"=w414) -> ("FrameColor"=w403:u32, "FrameThickness(1)"=w402:u32, "HeaderIcon"=w411:u8[][], "HeaderBkColor"=w412:u32, "BodyBkColor"=w404:u32, "error out"=w409:errorcluster)  [unwired: 5 in, 7 out]
            n184 = New VI(8:w409, 9:T4."Control VI" ("vi type (standard vi)"), 10:w445, 11:w397) -> (0:w448:errorcluster, 3:w447:refnum<vi>)  [unwired: 3 in]
            n185 = Build Array(w446) -> (w425:string[])
            n186 = property class="VI"(reference=w447, error in=w448, "Front Panel.Open"=FALSE ("Front Panel Window:Open")) -> (reference out=w401:refnum<vi>, error out=w435:errorcluster, "Panel"=w442:refnum<vi>)
            n187 = property class="Pnl"(reference=w442, error in=w435) -> (reference out=w429:refnum<vi>, error out=w436:errorcluster, "Controls[]"=w441:refnum<vi>[])
            n188 = Index Array(array=w441) -> (element=w440:refnum<vi>)  [unwired: 1 in]
            n189 = To More Specific Class(target class=w439, reference=w440, error in=w436) -> (specific class reference=w437:refnum<vi>, error out=w438:errorcluster)
            n190 = property class="TypRef"(reference=w437, error in=w438) -> (reference out=w431:refnum<vi>, error out=w432:errorcluster, "Element"=w433:refnum<vi>)
            n191 = To More Specific Class(target class=w434, reference=w433, error in=w432) -> (specific class reference=w427:refnum<vi>, error out=w426:errorcluster)
            n192 = property on="Ctrls" class="Enum"(reference=w427, error in=w426, "Strings []"=w425, "Named Numeric Colors:BG Color"=w412) -> (reference out=w424:refnum<vi>, error out=w423:errorcluster)
            n193 = Close Reference(reference=w424, error in (no error)=w423) -> (error out=w443:errorcluster)
            n194 = Close Reference(reference=w431, error in (no error)=w443) -> (error out=w430:errorcluster)
            n195 = Close Reference(reference=w429, error in (no error)=w430) -> (error out=w410:errorcluster)
            n196 = call <resource>:"GDSLvIcon_AnalyseViIcon.vi"("ViRef/LvCLassRef/LvLibRef/ViPath"=w401, "error in (no error)"=w410) -> ("BodyIcon"=w406:u8[][], "BodyBkColor"=w405:u32, "error out"=w407:errorcluster)  [unwired: 5 in, 10 out]
            n197 = call <resource>:"GDSLvIcon_ReplaceIconColor.vi"("IconIn"=w406, "OldColor"=w405, "NewColor"=w404, "error in (no error)"=w407) -> ("IconOut"=w408:u8[][])  [unwired: 14 in, 1 out]
            n198 = call <resource>:"GDSLvIcon_CreateIconPicture.vi"("FrameColor"=w403, "FrameThickness(1)"=w402, "HeaderIconIn"=w411, "BodyIconIn"=w408, "error in (no error)"=w409) -> ("WholeIconOut"=w420:u8[][], "error out"=w417:errorcluster)  [unwired: 9 in, 4 out]
            n199 = Reshape Array(w420, 1024 ("dimension size")) -> (w418:u8[])
            n200 = Bundle By Name(cluster=T3 {"image type"=0, "image depth"=8, "image"=[], "mask"=[], "colors"=[], "Rectangle"={"left"=0, "top"=0, "right"=32, "bottom"=32}} ("image data"), "image"=w418) -> (w421:T3)
            n201 = invoke class="VI" method="VI Icon.Set from Image Data"(reference=w401, error in=w417, "ImageData"=w421) -> (reference out=w416:refnum<vi>, error out=w415:errorcluster)  [unwired: 3 in, 4 out]
            n202 = invoke class="VI" method="Save.Instrument"(reference=w416, error in=w415, "Path to saved file"=w398) -> (reference out=w399:refnum<vi>, error out=w400:errorcluster)  [unwired: 3 in, 4 out]
          }
          frame True {
          }
        }
        n203 = Bundle By Name(cluster=w385, "SubObjectRef"=w384, "ObjectRef"=w386) -> (w388:T1)
      }
      frame "AddObjectRefToClass" {
        n204 = Unbundle By Name(w459) -> ("ObjectRef"=w451:refnum<vi>, "ThisSubClass"=w453:refnum<vi>, "SubObjectRef"=w454:path)
        n205 = Not A Number/Path/Refnum?(number/path/refnum=w451) -> (NaN/Path/Refnum?=w450:bool)
        n206 = case shown="False" w450 {
          tunnel: w457 -> [w469 w471]
          tunnel: [w462 w471] -> w456
          tunnel: w454 -> [w467 _]
          tunnel: w453 -> [w466 w472]
          tunnel: [w465 w472] -> w452
          tunnel: w451 -> [w464 _]
          frame False {
            n207 = invoke class="VI" method="Save.Instrument"(reference=w464, error in=w469, "Path to saved file"=w467) -> (reference out=w470:refnum<vi>, error out=w461:errorcluster)  [unwired: 3 in, 4 out]
            n208 = call <resource>:"CommonVIs_Wait.vi"("error in"=w461) -> ("error out"=w460:errorcluster)  [unwired: 9 in]
            n209 = Close Reference(reference=w470, error in (no error)=w460) -> (error out=w468:errorcluster)
            n210 = invoke class="LVClassLibrary" method="AddFile"(reference=w466, error in=w468, "Path"=w467) -> (reference out=w465:refnum<vi>, error out=w463:errorcluster)  [unwired: 1 in, 2 out]
            n211 = call <resource>:"CommonVIs_Wait.vi"("error in"=w463) -> ("error out"=w462:errorcluster)  [unwired: 9 in]
          }
          frame True {
          }
        }
        n212 = call <resource>:"GDSLvClass_SaveEverythingInClass.vi"("ClassRefIn"=w452, "error in"=w456) -> ("error out"=w455:errorcluster)  [unwired: 16 in, 1 out]
      }
      frame "ReplaceOldBaseObjectRefsWithNewRef" {
        n213 = Unbundle By Name(w488) -> ("AppRef"=w473:refnum<vi>, "AllSubClassFiles"=w491:path[], "RootObjectRef"=w492:path, "SubObjectRef"=w480:path, "ThisSubClass"=w486:refnum<vi>)
        n214 = property class="LVClassLibrary"(reference=w486, error in=w485) -> (reference out=w478:refnum<vi>, error out=w484:errorcluster, "Member Data"=w474:refnum<vi>)
        n215 = Build Array(w492) -> (w483:path[])
        n216 = for {
          tunnel: w483 -> [w515]
          tunnel: w491 -> [w514] mode=indexing
          shift-right: [w510] -> w487
          shift-left: w484 -> [w513]
          tunnel: [w507] -> w490 mode=indexing
          tunnel: w480 -> [w508]
          tunnel: w473 -> [w506]
          n217 = call <resource>:"Scripting_OpenViRef.vi"("error in"=w513, "ViPath/ViName/Viref"=w514, "AppRef"=w506) -> ("error out"=w512:errorcluster, "vi reference"=w507:refnum<vi>)  [unwired: 6 in, 1 out]
          n218 = call <resource>:"Scripting_FindControlsOnDiagram.vi"("ViRef"=w507, "TypeDefControlsToSerachFor"=w515, "error in (no error)"=w512) -> ("FronPanelControlsFound"=w509:refnum<vi>[], "error out"=w511:errorcluster)  [unwired: 14 in, 1 out]
          n219 = for {
            shift-right: [w516] -> w510
            shift-left: w511 -> [w520]
            tunnel: w509 -> [w522] mode=indexing
            tunnel: w508 -> [w521]
            n220 = invoke class="Ctl" method="Replace"(reference=w522, error in=w520, "Path"=w521) -> (reference out=w517:refnum<vi>, error out=w518:errorcluster, "Replace"=w519:refnum<vi>)  [unwired: 3 in, 3 out]
            n221 = Close Reference(reference=w517, error in (no error)=w518) -> ()  [unwired: 1 out]
            n222 = Close Reference(reference=w519, error in (no error)=w518) -> (error out=w516:errorcluster)
          }
        }
        n223 = call <resource>:"Scripting_FindControlsOnDiagram.vi"("ViRef"=w474, "TypeDefControlsToSerachFor"=w483, "error in (no error)"=w487) -> ("FronPanelControlsFound"=w481:refnum<vi>[], "error out"=w482:errorcluster)  [unwired: 14 in, 1 out]
        n224 = for {
          shift-right: [w493] -> w477
          shift-left: w482 -> [w497]
          tunnel: w481 -> [w499] mode=indexing
          tunnel: w480 -> [w498]
          n225 = invoke class="Ctl" method="Replace"(reference=w499, error in=w497, "Path"=w498) -> (reference out=w494:refnum<vi>, error out=w495:errorcluster, "Replace"=w496:refnum<vi>)  [unwired: 3 in, 3 out]
          n226 = Close Reference(reference=w494, error in (no error)=w495) -> ()  [unwired: 1 out]
          n227 = Close Reference(reference=w496, error in (no error)=w495) -> (error out=w493:errorcluster)
        }
        n228 = for {
          tunnel: w490 -> [w501] mode=indexing
          shift-right: [w505] -> w476
          shift-left: w477 -> [w502]
          n229 = call <resource>:"Scripting_SaveVi.vi"("ForceResaving(False)"=TRUE, "error in (no error)"=w502, "VIRefToSaveIn"=w501) -> ("error out"=w504:errorcluster, "VIRefToSaveOut"=w503:refnum<vi>)  [unwired: 7 in]
          n230 = Close Reference(reference=w503, error in (no error)=w504) -> (error out=w505:errorcluster)
        }
        n231 = invoke class="VI" method="Save.Instrument"(reference=w474, error in=w476) -> (error out=w475:errorcluster)  [unwired: 4 in, 5 out]
        n232 = invoke class="LVClassLibrary" method="Save"(reference=w478, error in=w475) -> (error out=w479:errorcluster)  [unwired: 2 in, 3 out]
        n233 = Close Reference(reference=w474, error in (no error)=w475) -> ()  [unwired: 1 out]
      }
      frame "RemoveInheritance" {
        # "Should we update the Class Template or not?"
        n234 = Unbundle By Name(w548) -> ("TemplateVersionUsed"=w526:string, "ThisSubClass"=w539:refnum<vi>)
        n235 = property class="LVClassLibrary"(reference=w539, error in=w538, "Parent"=refnum<vi> refnum ("Parent Class")) -> (reference out=w536:refnum<vi>, error out=w535:errorcluster)
        n236 = property class="LVClassLibrary"(reference=w539, error in=w538) -> ("Description"=w537:string)  [unwired: 2 out]
        n237 = call <resource>:"GDSLvClass_ReadClassType.vi"("Class Refnum In"=w536, "error in (no error)"=w535) -> ("Class Refnum Out"=w523:refnum<vi>, "ClassSettings"=w529:T9, "error out"=w534:errorcluster)  [unwired: 15 in]
        n238 = Unbundle By Name(w529) -> ("ClassTemplateUsed"=w525:string)
        n239 = Unbundle By Name(w529) -> ("ClassTemplateVersion"=w528:string)
        n240 = call <resource>:"GOOP_ClassTemplateSplit.vi"("ClassItemRefIn"=w523, "FullClassTemplate"=w525) -> ("StandardTemplate"=w524:string)  [unwired: 12 in, 1 out]
        n241 = case shown="True" w530 {
          tunnel: w524 -> [w557 w569]
          tunnel: [w553 w565] -> w532
          tunnel: [w552 w564] -> w531
          tunnel: w528 -> [w551 _]
          tunnel: [w551 w563] -> w527
          tunnel: w526 -> [_ w563]
          frame True {
            n242 = Scan From String(input string=w557, default 1=EndevoG4TemplateNames."G4SubTemplate_Simple_4x4x4" ("TemplateNames")) -> (output 1=w556:T5)  [unwired: 3 in, 3 out]
            n243 = case shown="\"G4SubTemplate_Singleton_6x8x6\"" w556 {
              tunnel: [EndevoG4TemplateNames."G4BaseTemplate_Simple_4x4x4" ("TemplateNames") EndevoG4TemplateNames."G4BaseTemplate_Simple_6x8x6" ("TemplateNames") EndevoG4TemplateNames."G4BaseTemplate_Singleton_4x4x4" ("TemplateNames") EndevoG4TemplateNames."G4BaseTemplate_Singleton_6x8x6" ("TemplateNames")] -> w555
              frame "G4SubTemplate_Simple_4x4x4", Default {
              }
              frame "G4SubTemplate_Simple_6x8x6" {
              }
              frame "G4SubTemplate_Singleton_4x4x4" {
              }
              frame "G4SubTemplate_Singleton_6x8x6" {
              }
            }
            n244 = Format Into String(EndevoG4ProviderName."EndevoGOOP400" ("ProviderName")) -> (resulting string=w553:string)  [unwired: 3 in, 1 out]
            n245 = Format Into String(w555) -> (resulting string=w552:string)  [unwired: 3 in, 1 out]
          }
          frame False {
            n246 = Scan From String(input string=w569, default 1=EndevoTemplateNames."SubTemplate" ("TemplateNames")) -> (output 1=w568:T7)  [unwired: 3 in, 3 out]
            n247 = case shown="\"SubTemplate_4x4x4\"" w568 {
              tunnel: [EndevoTemplateNames."BaseTemplate" ("TemplateNames") EndevoTemplateNames."BaseTemplate_4x4x4" ("TemplateNames")] -> w567
              frame "SubTemplate", Default {
              }
              frame "SubTemplate_4x4x4" {
              }
            }
            n248 = Format Into String(EndevoProviderName."EndevoGOOP300" ("ProviderName")) -> (resulting string=w565:string)  [unwired: 3 in, 1 out]
            n249 = Format Into String(w567) -> (resulting string=w564:string)  [unwired: 3 in, 1 out]
          }
        }
        n250 = Bundle By Name(cluster=w529, "ClassTemplateVersion"=w527, "ClassDescription"=w537, "ClassProviderName"=w532, "ClassTemplateUsed"=w531) -> (w542:T9)
        n251 = call <resource>:"GDSLvClass_StoreClassType.vi"("Class Refnum In"=w523, "ClassSettings"=w542, "error in (no error)"=w534) -> ("Class Refnum Out"=w541:refnum<vi>, "error out"=w540:errorcluster)  [unwired: 15 in]
        n252 = invoke class="LVClassLibrary" method="Save"(reference=w541, error in=w540) -> (reference out=w545:refnum<vi>, error out=w544:errorcluster)  [unwired: 2 in, 2 out]
        n253 = property class="LVClassLibrary"(reference=w545, error in=w544) -> (error out=w533:errorcluster, "Project"=w543:refnum<vi>)  [unwired: 1 out]
        n254 = invoke class="Project" method="Save"(reference=w543, error in=w533) -> (reference out=w546:refnum<vi>, error out=w547:errorcluster)  [unwired: 2 in, 2 out]
        n255 = Close Reference(reference=w546, error in (no error)=w547) -> ()  [unwired: 1 out]
      }
      frame "UpdateAllDerivedClasses" {
        n256 = case shown="False" w573 {
          tunnel: w578 -> [w581 w582]
          tunnel: [w580 w582] -> w577
          tunnel: w576 -> [w579 _]
          frame False {
            n257 = call <resource>:"Scripting_UpdateDerivedClasses.vi"("ClassRef"=w579, "error in (no error)"=w581) -> ("error out"=w580:errorcluster)  [unwired: 17 in]
          }
          frame True {
          }
        }
      }
      frame "UpdateNEWVI" {
        # "This is needed for GOOP4 templates"
        n258 = Unbundle By Name(w586) -> ("AppRef"=w583:refnum<vi>, "SubNewVi"=w585:path, "BaseNew"=w584:path)
        n259 = case shown="True" w589 {
          tunnel: w588 -> [w591 w596]
          tunnel: [w591 w595] -> w587
          tunnel: w585 -> [_ w594]
          tunnel: w584 -> [_ _]
          tunnel: w583 -> [_ w592]
          frame False {
          }
          frame True {
            w593 = path ""  # Leave emptysince no base class should be used
            n260 = call <resource>:"Scripting_UpdateNewVI.vi"("NewVI Ref or Path"=w594, "BaseClassNewVI Ref or Path(If empty the No base class will be used)"=w593, "error in (no error)"=w596, "AppRef"=w592) -> ("error out"=w595:errorcluster)  [unwired: 15 in]
          }
        }
      }
      frame "CloseReferences", "Error", Default {
        n261 = call <resource>:"GDSError_LogErrorInformation.vi"("State"=w599, "LocalVariableData"=w598, "error in (no error)"=w597) -> ()  [unwired: 16 in, 1 out]
        n262 = Unbundle By Name(w598) -> ("CurrentBaseClass"=w601:refnum<vi>)  [unwired: 2 out]
        n263 = Close Reference(reference=w601) -> ()  [unwired: 1 in, 1 out]
      }
    }
    n264 = Equal?(x=w14, y="Exit") -> (x = y?=w17:bool)
    n265 = Select(t="Error", s=w13, f=w14) -> (s? t:f=w18:string)
  }
  "error out" <- w5
